vi "Create Battery Control.vi"(8 "error in (no error)":errorcluster, 11 "Device Item Ref in":T1 format="%.0x") -> (0 "error out":errorcluster)   [LabVIEW 2021, in "G5 Regatron Custom Device System Explorer.lvlib"]
doc: "Creates folder in custom device with battery control channels"
uses:
  G5 Regatron Custom Device System Explorer.lvlib
  <vilib>/NI VeriStand/Custom Device API/Custom Device Item Ref.ctl
  <vilib>/NI VeriStand/Custom Device API/Custom Device Channel.ctl
  <vilib>/NI VeriStand/Custom Device API/Custom Device Channel Type.ctl
  <vilib>/NI VeriStand/Custom Device API/Custom Device API.lvlib
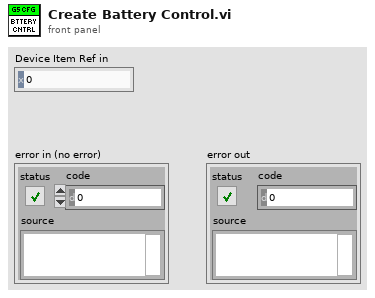
[diagram p1: front panel]
types:
  T1 = typedef "Custom Device API.lvlib/Custom Device Item Ref.ctl" = u64
  T2 = typedef "Custom Device API.lvlib/Custom Device Channel.ctl" = cluster{"Type":T3, "Units":string, "Default Value":dbl, "Faultable":bool, "Scalable":bool}
  T3 = typedef "Custom Device API.lvlib/Custom Device Channel Type.ctl" = enum16{"Input", "Output"}
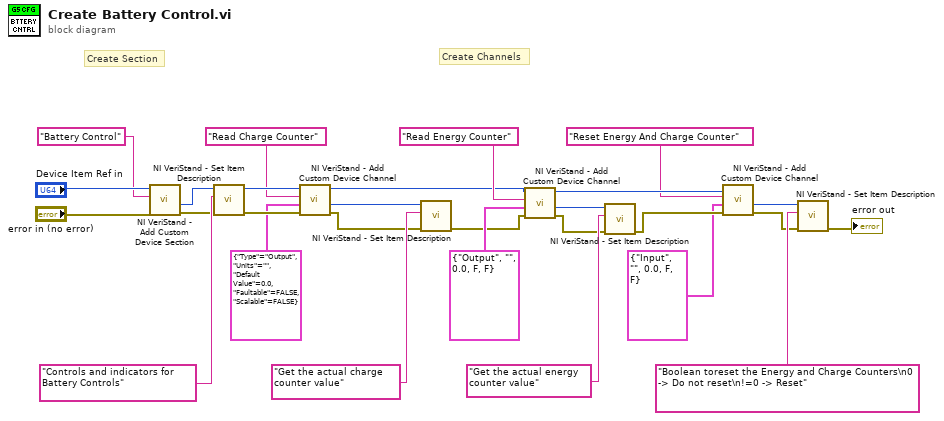
[diagram p0: block diagram]
diagram:
  # "Create Channels"
  # "Create Section"
  n1 = call <vilib>:"NI VeriStand - Add Custom Device Section.vi"("error in (no error)"="error in (no error)", "Section Name"="Battery Control", "Parent Ref in"="Device Item Ref in") -> ("error out"=w13:errorcluster, "Section Ptr"=w15:T1)  [unwired: 5 in, 2 out]
  n2 = call <vilib>:"NI VeriStand - Set Item Description.vi"("error in (no error)"=w13, "Description"="Controls and indicators for Battery Controls", "Item Ref in"=w15) -> ("error out"=w14:errorcluster, "Item Ref out"=w16:T1)  [unwired: 6 in, 1 out]
  n3 = call <vilib>:"NI VeriStand - Add Custom Device Channel.vi"("error in (no error)"=w14, "Channel"=T2 {"Type"=enum."Output", "Units"="", "Default Value"=0.0, "Faultable"=FALSE, "Scalable"=FALSE}, "Channel Name"="Read Charge Counter", "Parent Ref in"=w16) -> ("error out"=w8:errorcluster, "Channel Ref"=w7:T1, "Parent Ref out"=w20:T1)  [unwired: 4 in, 1 out]
  n4 = call <vilib>:"NI VeriStand - Set Item Description.vi"("error in (no error)"=w8, "Description"="Get the actual charge counter value", "Item Ref in"=w7) -> ("error out"=w22:errorcluster)  [unwired: 6 in, 2 out]
  n5 = call <vilib>:"NI VeriStand - Add Custom Device Channel.vi"("error in (no error)"=w22, "Channel"=T2 {"Type"=enum."Output", "Units"="", "Default Value"=0.0, "Faultable"=FALSE, "Scalable"=FALSE}, "Channel Name"="Read Energy Counter", "Parent Ref in"=w20) -> ("error out"=w25:errorcluster, "Channel Ref"=w24:T1, "Parent Ref out"=w21:T1)  [unwired: 4 in, 1 out]
  n6 = call <vilib>:"NI VeriStand - Set Item Description.vi"("error in (no error)"=w25, "Description"="Get the actual energy counter value", "Item Ref in"=w24) -> ("error out"=w26:errorcluster)  [unwired: 6 in, 2 out]
  n7 = call <vilib>:"NI VeriStand - Add Custom Device Channel.vi"("error in (no error)"=w26, "Channel"=T2 {"Type"=enum."Input", "Units"="", "Default Value"=0.0, "Faultable"=FALSE, "Scalable"=FALSE}, "Channel Name"="Reset Energy And Charge Counter", "Parent Ref in"=w21) -> ("error out"=w10:errorcluster, "Channel Ref"=w11:T1)  [unwired: 4 in, 2 out]
  n8 = call <vilib>:"NI VeriStand - Set Item Description.vi"("error in (no error)"=w10, "Description"="Boolean toreset the Energy and Charge Counters\n0 -> Do not reset\n!=0 -> Reset", "Item Ref in"=w11) -> ("error out"=→"error out":errorcluster)  [unwired: 6 in, 2 out]
